vi "Send email notice.vi"(8 "error in (no error)":errorcluster, 10 "Notice type":T1=enum."Tomography error", 11 "Tomo in":refnum<class "Tomo.lvclass">) -> (0 "error out":errorcluster, 3 "Tomo out":refnum<class "Tomo.lvclass">)   [LabVIEW 2012, in "Tomo.lvclass"]
uses:
  Tomo.lvclass
  notice type.ctl
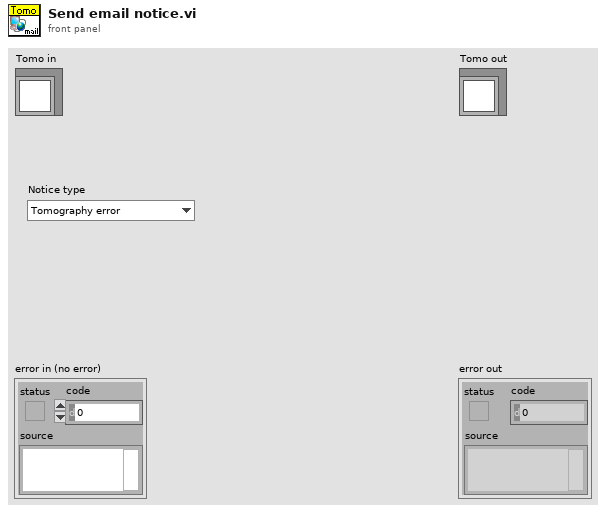
[diagram p1: front panel]
types:
  T1 = typedef "Tomo.lvclass/notice type.ctl" = enum16{"Tomography stopped", "Tomography error", "Tomography finished", "Timing issue", "Critical timing issue"}
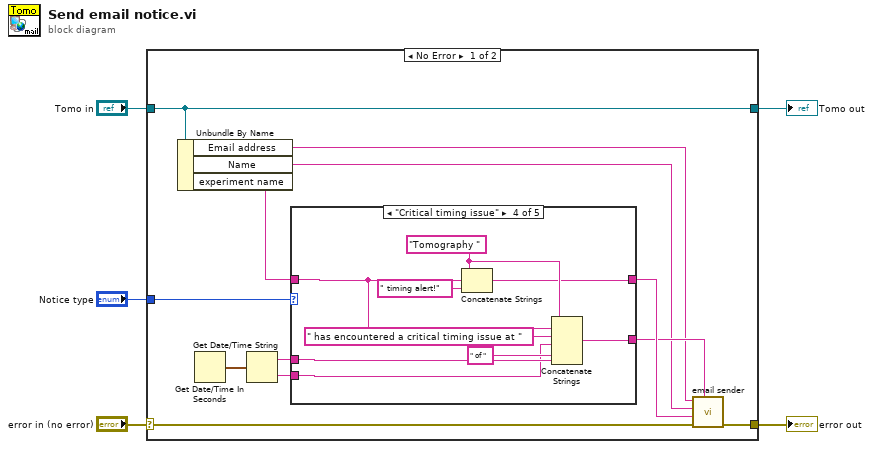
[diagram p0: block diagram]
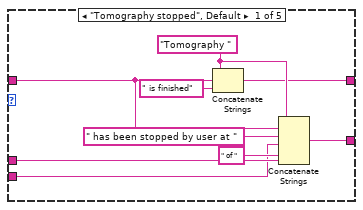
[diagram p2: hidden frame]
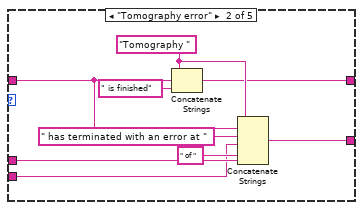
[diagram p3: hidden frame]
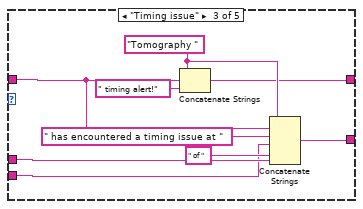
[diagram p4: hidden frame]
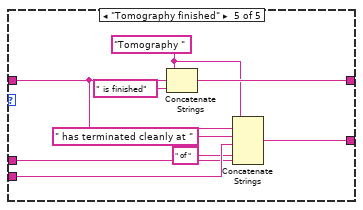
[diagram p5: hidden frame]
diagram:
  n1 = case shown="No Error" "error in (no error)" {
    selector: "error in (no error)" -> [w7 w64]
    tunnel: [w6 w64] -> w4
    tunnel: [w17 w63] -> w2
    tunnel: "Tomo in" -> [w17 w63]
    tunnel: "Notice type" -> [w16 _]
    frame No Error {
      n2 = Unbundle By Name(w17) -> ("Email address"=w9:string, "Name"=w8:string, "experiment name"=w15:string)
      n3 = Get Date/Time In Seconds() -> (seconds since 1Jan1904=w13:timestamp)
      n4 = Get Date/Time String(seconds (now)=w13) -> (date string=w11:string, time string=w12:string)  [unwired: 2 in]
      n5 = case shown="\"Critical timing issue\"" w16 {
        tunnel: w15 -> [w20 w29 w40 w49 w59]
        tunnel: [w18 w30 w37 w46 w61] -> w14
        tunnel: w12 -> [w21 w27 w38 w47 w57]
        tunnel: w11 -> [w22 w28 w39 w48 w55]
        tunnel: [w19 w31 w36 w45 w54] -> w10
        frame "Tomography stopped", Default {
          w25 = "Tomography " ("string")
          n6 = Concatenate Strings(w25, w20, " is finished" ("string")) -> (w18:string)
          n7 = Concatenate Strings(w25, w20, " has been stopped by user at " ("string"), w21, " of " ("string"), w22) -> (w19:string)
        }
        frame "Tomography error" {
          w33 = "Tomography " ("string")
          n8 = Concatenate Strings(w33, w29, " is finished" ("string")) -> (w30:string)
          n9 = Concatenate Strings(w33, w29, " has terminated with an error at " ("string"), w27, " of " ("string"), w28) -> (w31:string)
        }
        frame "Timing issue" {
          w42 = "Tomography " ("string")
          n10 = Concatenate Strings(w42, w40, " timing alert!" ("string")) -> (w37:string)
          n11 = Concatenate Strings(w42, w40, " has encountered a timing issue at " ("string"), w38, " of " ("string"), w39) -> (w36:string)
        }
        frame "Critical timing issue" {
          w51 = "Tomography " ("string")
          n12 = Concatenate Strings(w51, w49, " timing alert!" ("string")) -> (w46:string)
          n13 = Concatenate Strings(w51, w49, " has encountered a critical timing issue at " ("string"), w47, " of " ("string"), w48) -> (w45:string)
        }
        frame "Tomography finished" {
          w60 = "Tomography " ("string")
          n14 = Concatenate Strings(w60, w59, " is finished" ("string")) -> (w61:string)
          n15 = Concatenate Strings(w60, w59, " has terminated cleanly at " ("string"), w57, " of " ("string"), w55) -> (w54:string)
        }
      }
      n16 = call "email sender.vi"("Body"=w10, "error in (no error)"=w7, "Subject"=w14, "Recipient's Name"=w8, "Recipient's Email Address Address"=w9) -> ("error out"=w6:errorcluster)  [unwired: 6 in]
    }
    frame Error {
    }
  }
  "error out" <- w4
  "Tomo out" <- w2
